vi "Msg.vi"(7 "Actor in":refnum<class "Actor.lvclass">, 11 "TEMPLATE Msg Strategy in":refnum<class "TEMPLATE Msg Strategy.lvclass">) -> (5 "Actor out":refnum<class "Actor.lvclass">)   [LabVIEW 2021, in "_Template.lvlib" / "Templates.lvlib" / "TEMPLATE Msg Strategy.lvlib" / "TEMPLATE Msg Strategy.lvclass"]
uses:
  TEMPLATE Msg Strategy.lvclass
  TEMPLATE Msg Strategy.lvclass/TEMPLATE Msg Strategy.ctl
  TEMPLATE/TEMPLATE.lvclass
  jettl/jettl/Actor/Actor/Actor.lvclass
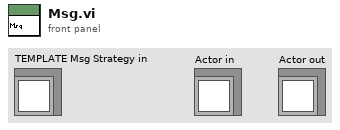
[diagram p1: front panel]
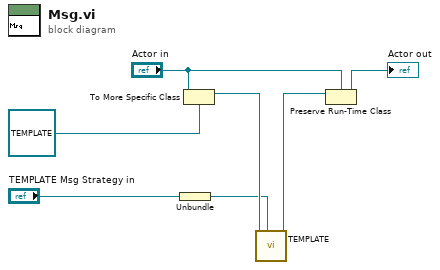
[diagram p0: block diagram]
diagram:
  n1 = Unbundle "Unbundle"("TEMPLATE Msg Strategy in") -> (w3:refnum<class "Sender.lvclass">)
  n2 = To More Specific Class(target class=refnum<class "TEMPLATE.lvclass"> refnum ("jettl Msg Template"), reference="Actor in") -> (specific class reference=w5:refnum<class "TEMPLATE.lvclass">)  [unwired: 1 in, 1 out]
  n3 = call-dynamic "TEMPLATE.vi"("Sender"=w3, "TEMPLATE in"=w5) -> ("TEMPLATE out"=w4:refnum<class "TEMPLATE.lvclass">)  [unwired: 9 in]
  n4 = Preserve Run-Time Class(object in=w4, 2:"Actor in") -> (object out=→"Actor out":refnum<class "Actor.lvclass">)  [unwired: 1 in, 1 out]
